vi "Get Variables.vi"(8 "error in (no error)":errorcluster, 11 "For Loop in":refnum<class "For Loop.lvclass">) -> (0 "error out":errorcluster, 2 "Variables":variant, 3 "For Loop out":refnum<class "For Loop.lvclass">)   [LabVIEW 2016, in "For Loop.lvclass"]
uses:
  For Loop.lvclass
  For Loop.lvclass/For Loop.ctl
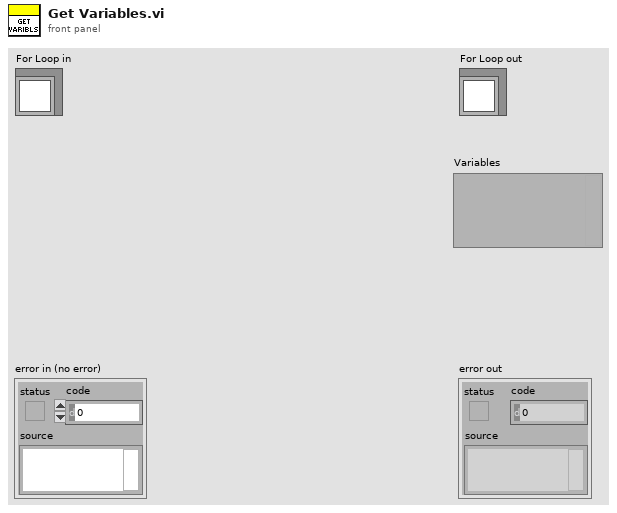
[diagram p1: front panel]
types:
  T1 = typedef "For Loop.lvclass/Variables.ctl" = cluster{"Start":dbl, "Stop":dbl, "Step":dbl}
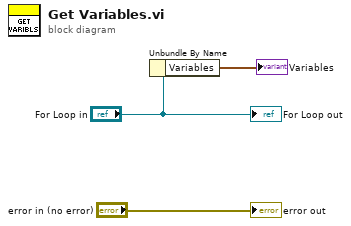
[diagram p0: block diagram]
diagram:
  n1 = Unbundle By Name("For Loop in") -> ("Variables"=→"Variables":T1)
  "error out" <- "error in (no error)"
  "For Loop out" <- "For Loop in"
